vi "自动升级更新main.vi"() -> ()   [LabVIEW 2016, in "数据传输系统-04.lvlib" / "自动更新.lvlib"]
panel:
  out "waittime":u8
  out "有新版本":bool
  out "下载的文件名":string
  out "最新版本获取进度":u8(slide) scale=0.0..100.0
  # "版本获取中，请稍后！"
  # "s"
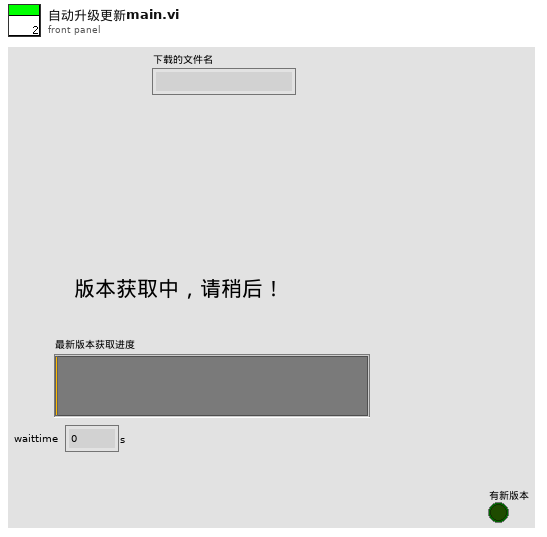
[diagram p1: front panel]
types:
  T1 = enum16{"get version information", "get success", "contact", "over"}
  T2 = cluster{"网络灯":bool, "接收中":bool, "已接收百分比":u8, "接收成功次数":dbl, "当前步骤":enum16{"init", "receivehead", "receivecontent", "receivesuccess", "over"}, "文件名":string, "error out":errorcluster}
  T3 = enum16{"open", "replace", "create", "open or create", "replace or create", "replace or create with confirmation"}
  T4 = enum32{"Bad", "Idle", "Run top level", "Running"}
  T5 = cluster{"主机":string, "用户":string, "密码":string, "远程路径":string, "下载文件名":string, "软件版本":string}
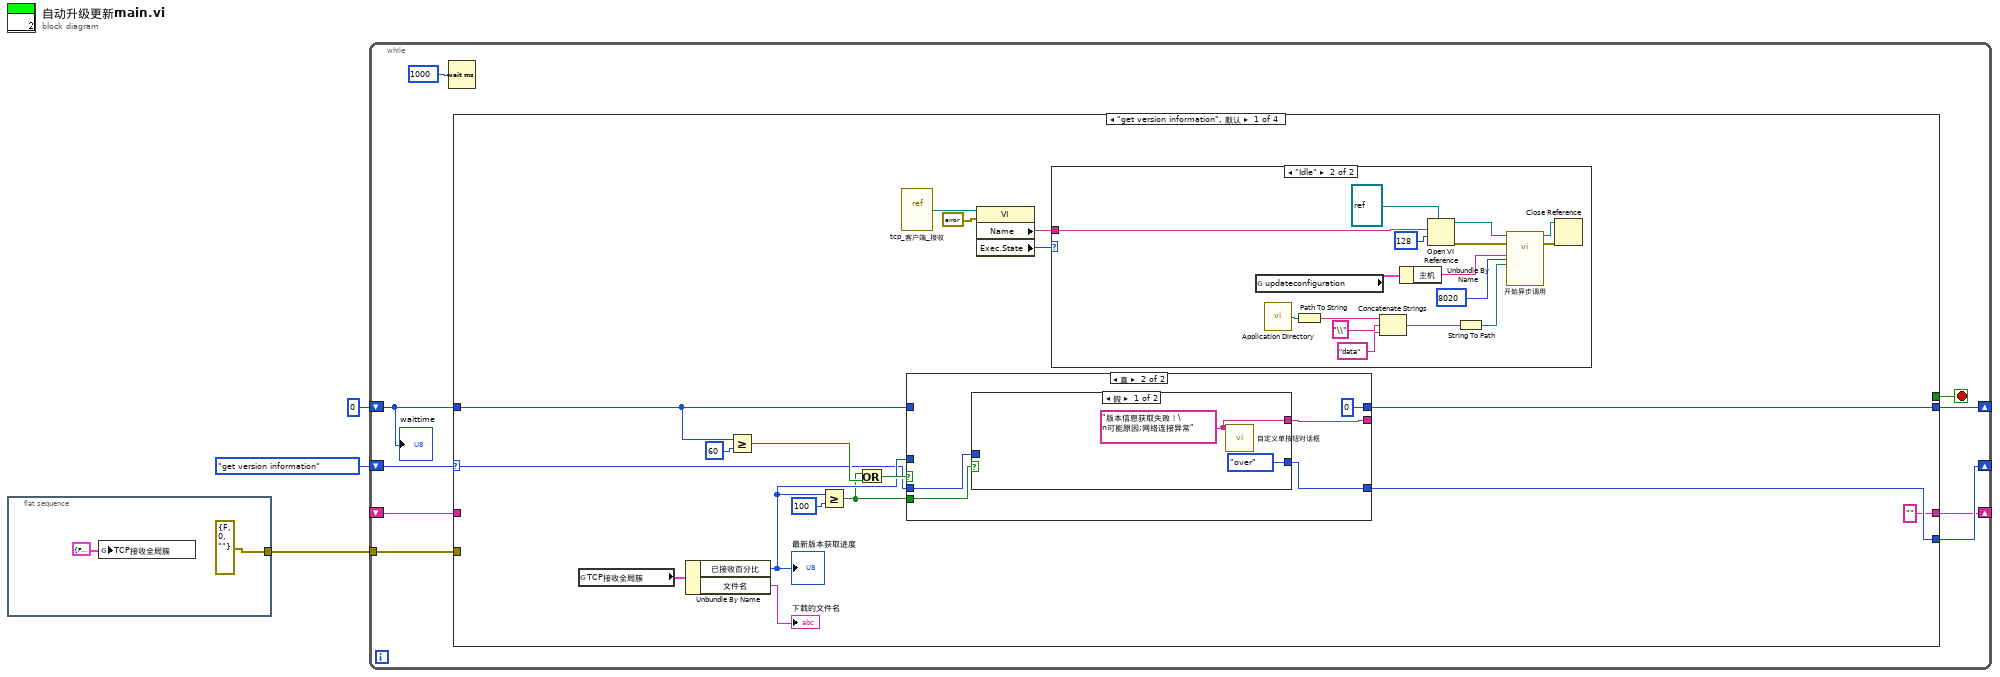
[diagram p0: block diagram]
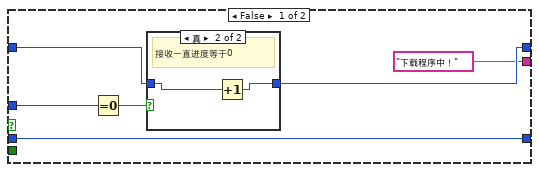
[diagram p2: hidden frame]
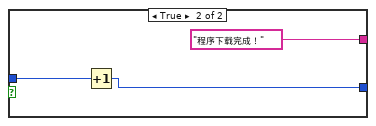
[diagram p4: hidden frame]
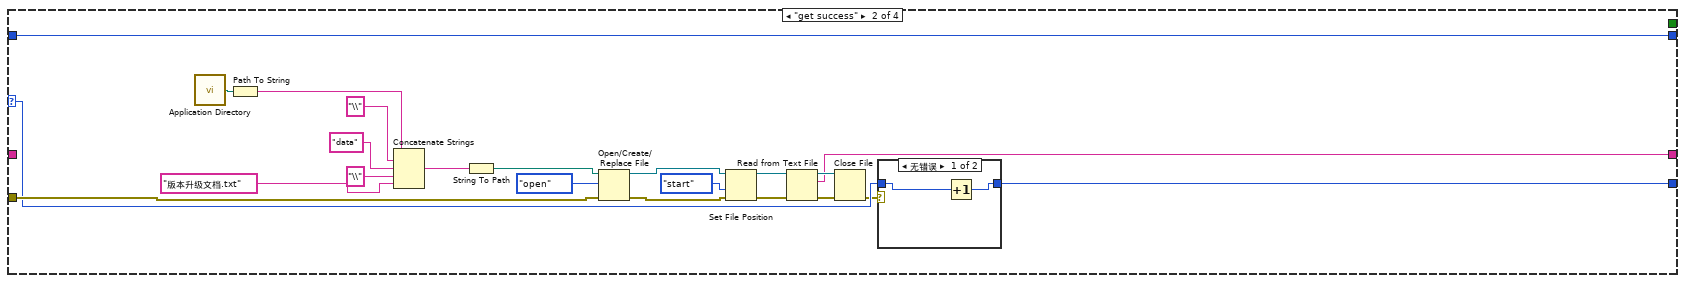
[diagram p6: hidden frame]
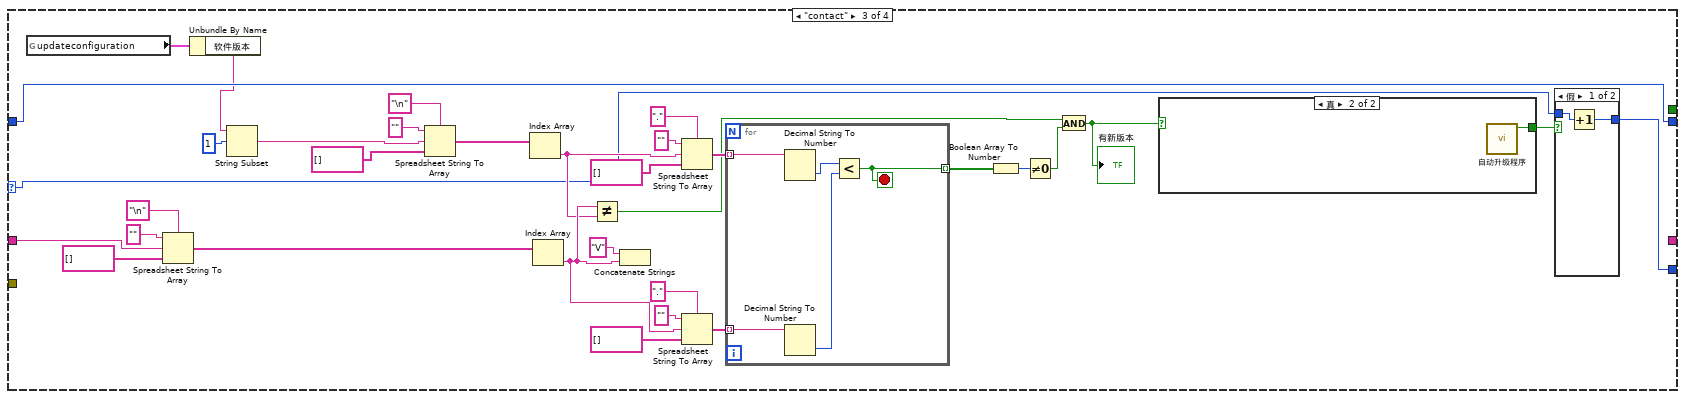
[diagram p8: hidden frame]
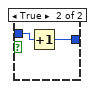
[diagram p9: hidden frame]
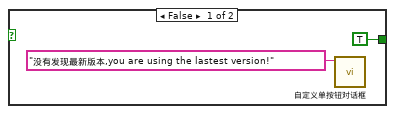
[diagram p10: hidden frame]
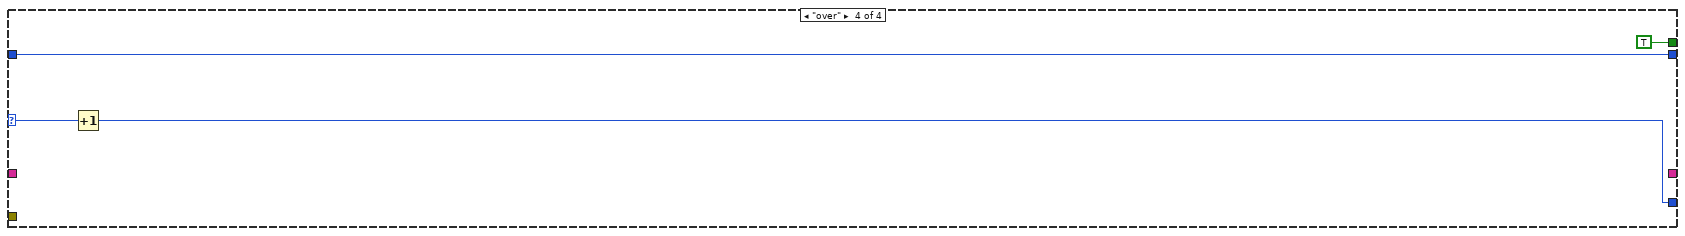
[diagram p11: hidden frame]
diagram:
  n1 = flat-sequence {
    tunnel: [errorcluster {"status"=FALSE, "code"=0, "source"=""} ("错误常量")] -> w1
    frame #0 {
      n2 = global write "全局变量1.vi" "TCP接收全局簇"(T2 {"网络灯"=FALSE, "接收中"=FALSE, "已接收百分比"=0, "接收成功次数"=0.0, "当前步骤"=enum."init", "文件名"="", "error out"={"status"=FALSE, "code"=0, "source"=""}} ("TCP接收全局簇")) -> ()
    }
  }
  n3 = while {
    shift-right: [w10] -> _
    shift-left: T1."get version information" -> [w13]
    shift-right: [w11] -> _
    shift-left: u8 0 ("y") -> [w12]
    tunnel: w1 -> [w9]
    shift-right: [w8] -> _
    shift-left: _ -> [w7]
    stop <- w6 stop-if-true
    n4 = Wait (ms)(milliseconds to wait=u32 1000 ("等待时间（毫秒）")) -> ()  [unwired: 1 out]
    n5 = case shown="\"get version information\", 默认" w13 {
      selector: w13 -> [w17 w75 w96 w138]
      tunnel: w12 -> [w19 w67 w94 w139]
      tunnel: [w18 w67 w94 w139] -> w11
      tunnel: [w16 w74 w95 w137] -> w10
      tunnel: w9 -> [_ w76 _ _]
      tunnel: ["" w68 _ _] -> w8
      tunnel: w7 -> [_ _ w99 _]
      tunnel: [_ _ _ TRUE] -> w6
      frame "get version information", Default {
        n6 = global read "全局变量1.vi" "TCP接收全局簇"() -> (w22:T2)
        n7 = Unbundle By Name(w22) -> ("已接收百分比"=w23:u8, "文件名"=→"下载的文件名":string)
        "最新版本获取进度" <- w23
        n8 = Greater Or Equal?(x=w19, y=u8 60) -> (x >= y?=w25:bool)
        n9 = Greater Or Equal?(x=w23, y=u8 100) -> (x >= y?=w21:bool)
        n10 = Or(x=w21, y=w25) -> (x .or. y?=w24:bool)
        n11 = vi-ref "tcp_客户端_接收.vi"() -> (w31:refnum<vi>)
        n12 = case shown="真" w24 {
          tunnel: w19 -> [w37 _]
          tunnel: [w36 u8 0] -> w18
          tunnel: w23 -> [w34 _]
          tunnel: [w33 w41] -> w16
          tunnel: w17 -> [w33 w42]
          tunnel: ["下载程序中！" w43] -> _
          tunnel: w21 -> [_ w44]
          frame False {
            n13 = Equal To 0?(x=w34) -> (x = 0?=w35:bool)
            n14 = case shown="真" w35 {
              tunnel: w37 -> [w38 w40]
              tunnel: [w38 w39] -> w36
              frame False {
              }
              frame True {
                # "接收一直进度等于0"
                n15 = Increment(x=w40) -> (x+1=w39:u8)
              }
            }
          }
          frame True {
            n16 = case shown="假" w44 {
              tunnel: [w47 "程序下载完成！"] -> w43
              tunnel: w42 -> [_ w49]
              tunnel: [T1."over" w48] -> w41
              frame False {
                w47 = "版本信息获取失败！\n可能原因;网络连接异常"
                n17 = call "自定义单按钮对话框.vi"("消息"=w47) -> ()  [unwired: 11 in]
              }
              frame True {
                n18 = Increment(x=w49) -> (x+1=w48:T1)
              }
            }
          }
        }
        n19 = property class="VI"(reference=w31, error in=errorcluster {"status"=FALSE, "code"=0, "source"=""} ("错误输出")) -> ("Name"=w30:string, "Exec.State"=w28:T4)  [unwired: 2 out]
        n20 = case shown="\"Idle\"" w28 {
          tunnel: w30 -> [_ w66]
          frame "Bad", Default {
          }
          frame "Idle" {
            n21 = global read "update全局.vi" "updateconfiguration"() -> (w59:T5)
            n22 = call <vilib>:"Application Directory.vi"() -> ("Application Directory"=w56:path)
            n23 = Path To String(path=w56) -> (string=w53:string)
            n24 = Concatenate Strings(w53, "\\" ("字符串"), "data" ("字符串")) -> (w57:string)
            n25 = Unbundle By Name(w59) -> ("主机"=w58:string)
            n26 = Open VI Reference(type specifier VI Refnum (for type only)=refnum<vi> refnum, vi path=w66, options=128 ("选项")) -> (vi reference=w64:refnum<vi>, error out=w62:errorcluster)  [unwired: 3 in]
            n27 = String To Path(string=w57) -> (path=w52:path)
            n28 = call-by-ref "开始异步调用"(reference=w64, error in=w62, "IP地址"=w58, "端口号"=8020, "储存路径"=w52) -> (reference out=w60:refnum<vi>, error out=w61:errorcluster)  [unwired: 17 in]
            n29 = Close Reference(reference=w60, error in (no error)=w61) -> ()  [unwired: 1 out]
          }
        }
      }
      frame "get success" {
        n30 = call <vilib>:"Application Directory.vi"() -> ("Application Directory"=w81:path)
        n31 = Path To String(path=w81) -> (string=w84:string)
        n32 = Concatenate Strings(w84, "\\" ("字符串"), "data" ("字符串"), "\\" ("字符串"), "版本升级文档.txt" ("字符串")) -> (w78:string)
        n33 = String To Path(string=w78) -> (path=w77:path)
        n34 = Open/Create/Replace File(file path (use dialog)=w77, error in=w76, operation (0:open)=T3."open" ("操作(0:open)")) -> (refnum out=w87:refnum<file>, error out=w86:errorcluster)  [unwired: 3 in, 1 out]
        n35 = Set File Position(refnum=w87, from (0:start)=enum16{"start", "end", "current"}."start" ("自（0:起始）"), error in=w86) -> (refnum out=w72:refnum<file>, error out=w71:errorcluster)  [unwired: 1 in]
        n36 = Read from Text File(file (use dialog)=w72, error in=w71) -> (refnum out=w73:refnum<file>, text=w68:string, error out=w70:errorcluster)  [unwired: 2 in, 1 out]
        n37 = Close File(refnum=w73, error in=w70) -> (error out=w69:errorcluster)  [unwired: 1 out]
        n38 = case shown="无错误" w69 {
          tunnel: w75 -> [w90 w91]
          tunnel: [w89 w91] -> w74
          frame No Error {
            n39 = Increment(x=w90) -> (x+1=w89:T1)
          }
          frame Error {
          }
        }
      }
      frame "contact" {
        n40 = global read "update全局.vi" "updateconfiguration"() -> (w93:T5)
        n41 = Spreadsheet String To Array(delimiter (Tab)="\n" ("分隔符(Tab)"), format string="" ("格式字符串"), spreadsheet string=w99, array type (2D Dbl)=string[] []) -> (array=w120:string[])
        n42 = Unbundle By Name(w93) -> ("软件版本"=w92:string)
        n43 = String Subset(string=w92, offset (0)=1 ("偏移量(0)")) -> (substring=w112:string)  [unwired: 1 in]
        n44 = Spreadsheet String To Array(delimiter (Tab)="\n" ("分隔符(Tab)"), format string="" ("格式字符串"), spreadsheet string=w112, array type (2D Dbl)=string[] []) -> (array=w111:string[])
        n45 = Index Array(array=w111) -> (element=w102:string)  [unwired: 1 in]
        n46 = Index Array(array=w120) -> (element=w103:string)  [unwired: 1 in]
        n47 = Not Equal?(x=w103, y=w102) -> (x != y?=w100:bool)
        n48 = Concatenate Strings("V" ("字符串"), w103) -> ()  [unwired: 1 out]
        n49 = Spreadsheet String To Array(delimiter (Tab)="." ("分隔符(Tab)"), format string="" ("格式字符串"), spreadsheet string=w102, array type (2D Dbl)=string[] []) -> (array=w106:string[])
        n50 = Spreadsheet String To Array(delimiter (Tab)="." ("分隔符(Tab)"), format string="" ("格式字符串"), spreadsheet string=w103, array type (2D Dbl)=string[] []) -> (array=w107:string[])
        n51 = for {
          tunnel: w107 -> [w134] mode=indexing
          tunnel: w106 -> [w136] mode=indexing
          tunnel: [w135] -> w105 mode=indexing
          stop <- w135 stop-if-true
          n52 = Decimal String To Number(string=w136) -> (number=w133:i32)  [unwired: 2 in, 1 out]
          n53 = Decimal String To Number(string=w134) -> (number=w132:i32)  [unwired: 2 in, 1 out]
          n54 = Less?(x=w133, y=w132) -> (x < y?=w135:bool)
        }
        n55 = Boolean Array To Number(Boolean array=w105) -> (number=w104:u32)
        n56 = Not Equal To 0?(x=w104) -> (x != 0?=w101:bool)
        n57 = And(x=w100, y=w101) -> (x .and. y?=w98:bool)
        "有新版本" <- w98
        n58 = case shown="真" w98 {
          tunnel: [TRUE ("确定") w131] -> w97
          frame False {
            n59 = call "自定义单按钮对话框.vi"("消息"="没有发现最新版本,you are using the lastest version!") -> ()  [unwired: 11 in]
          }
          frame True {
            n60 = call "自动升级程序.vi"() -> ("确定"=w131:bool)  [unwired: 10 in, 1 out]
          }
        }
        n61 = case shown="假" w97 {
          tunnel: w96 -> [w126 w128]
          tunnel: [w125 w127] -> w95
          frame False {
            n62 = Increment(x=w126) -> (x+1=w125:T1)
          }
          frame True {
            n63 = Increment(x=w128) -> (x+1=w127:T1)
          }
        }
      }
      frame "over" {
        n64 = Increment(x=w138) -> (x+1=w137:T1)
      }
    }
    "waittime" <- w12
  }
